vi "GetPositionValue.vi"(1 "DesiredPosition":T1, 2 "Climb Heights":T2) -> (0 "PositionHeight":dbl)   [LabVIEW 2018]
uses:
  TypeDefs/ClimberPositionHeights.ctl
  TypeDefs/ClimberPositions.ctl
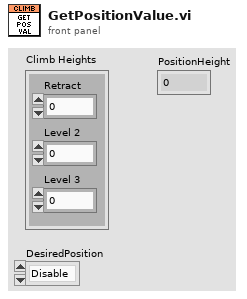
[diagram p1: front panel]
types:
  T1 = typedef "ClimberPositions.ctl" = enum16{"Disable", "Floor", "Level 2", "Level 3"}
  T2 = typedef "ClimberPositionHeights.ctl" = cluster{"Retract":dbl, "Level 2":dbl, "Level 3":dbl}
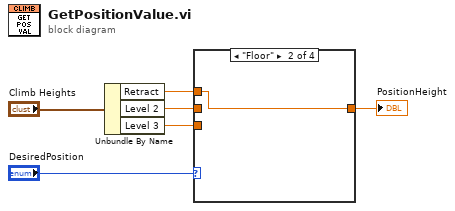
[diagram p0: block diagram]
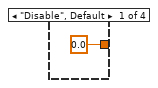
[diagram p2: hidden frame]
diagram:
  n1 = Unbundle By Name("Climb Heights") -> ("Retract"=w4:dbl, "Level 2"=w3:dbl, "Level 3"=w2:dbl)
  n2 = case shown="\"Floor\"" "DesiredPosition" {
    tunnel: w4 -> [_ w8 _ _]
    tunnel: w3 -> [_ _ w9 _]
    tunnel: w2 -> [_ _ _ w10]
    tunnel: [0.0 ("Level 3") w8 w9 w10] -> w1
    frame "Disable", Default {
    }
    frame "Floor" {
    }
    frame "Level 2" {
    }
    frame "Level 3" {
    }
  }
  "PositionHeight" <- w1
